vi "STC_main_raw_1.vi"() -> ()   [LabVIEW 2017]
uses:
  controls/FPGA State.ctl
  controls/UI Data2.ctl
  controls/Chatter data.ctl
  Globals/Global - All UI Loop Stop.vi
  Globals/Global - UI Stream and Variable Connections.vi
  Globals/Global - Configuration Options.vi
  UI Error Handlers/support/User Event - Stop/User Event - Stop.lvlib
  UI Error Handlers/support/Message Queue/Message Queue.lvlib
panel:
  out "resulting string":string
  out "Raw Waveform":waveform(dbl)[](graph)
  in  "Settings Tab":T1(tab)=enum."Data Monitoring"
  in  "OK Button":bool
  in  "Tool Data File":path=path "K:/Core Research/Project Folders/AI Projects/AI3190 Digital Shop Floor Rollout/5 Software Files/Catapult/tool_path.txt"
  in  "Run Control":bool
  in  "Stop Control":bool
  in  "Max Acceleration Threshold (g)":sgl=0.03
  in  "In-cut Power Threshold":dbl=1.0
  in  "Controller Address":string="172.22.11.2"
  in  "Connect to Controller":bool
  out "Connected?":bool
  out "System Status":string
  in  "Save?":bool
  in  "Switch to Safe State":bool
  out "Current FPGA State":T2
  out "Tool Data":string="\n"
  in  "ODBC data source name":string="amrc_monitoring"
  in  "MT Connect Agent":string="http://amrcmtconnect.shef.ac.uk:5000/"
  in  "milliseconds to wait":u32=100
  in  "Machine":string="STC1250"
  out "Loop execution":u32
  out "output cluster":cluster{"G1 ":bool}
  out "tag acc":string
  out "tag spike":string
  out "Chatter?":bool
  out "Feed":dbl
  out "ACC  (grms)":T3(graph)
  out "Block of code being executed":string
  out "Program Name":string
  out "RPM":dbl
  out "STC Starrag":bool
  out "Force (grms)":T4(graph)
  out "Tool id":string
  out "Spindle Load":dbl[](graph)
  out "CPU Usage (%)":dbl[][](graph)
  out "Free Physical Memory or Largest Contiguous Memory (bytes)":dbl(graph)
  out "DMA FIFO Overflow?":bool
  in  "Exit":bool
  # "Acceleration Waveform for 0.5s"
  # "Connection Settings"
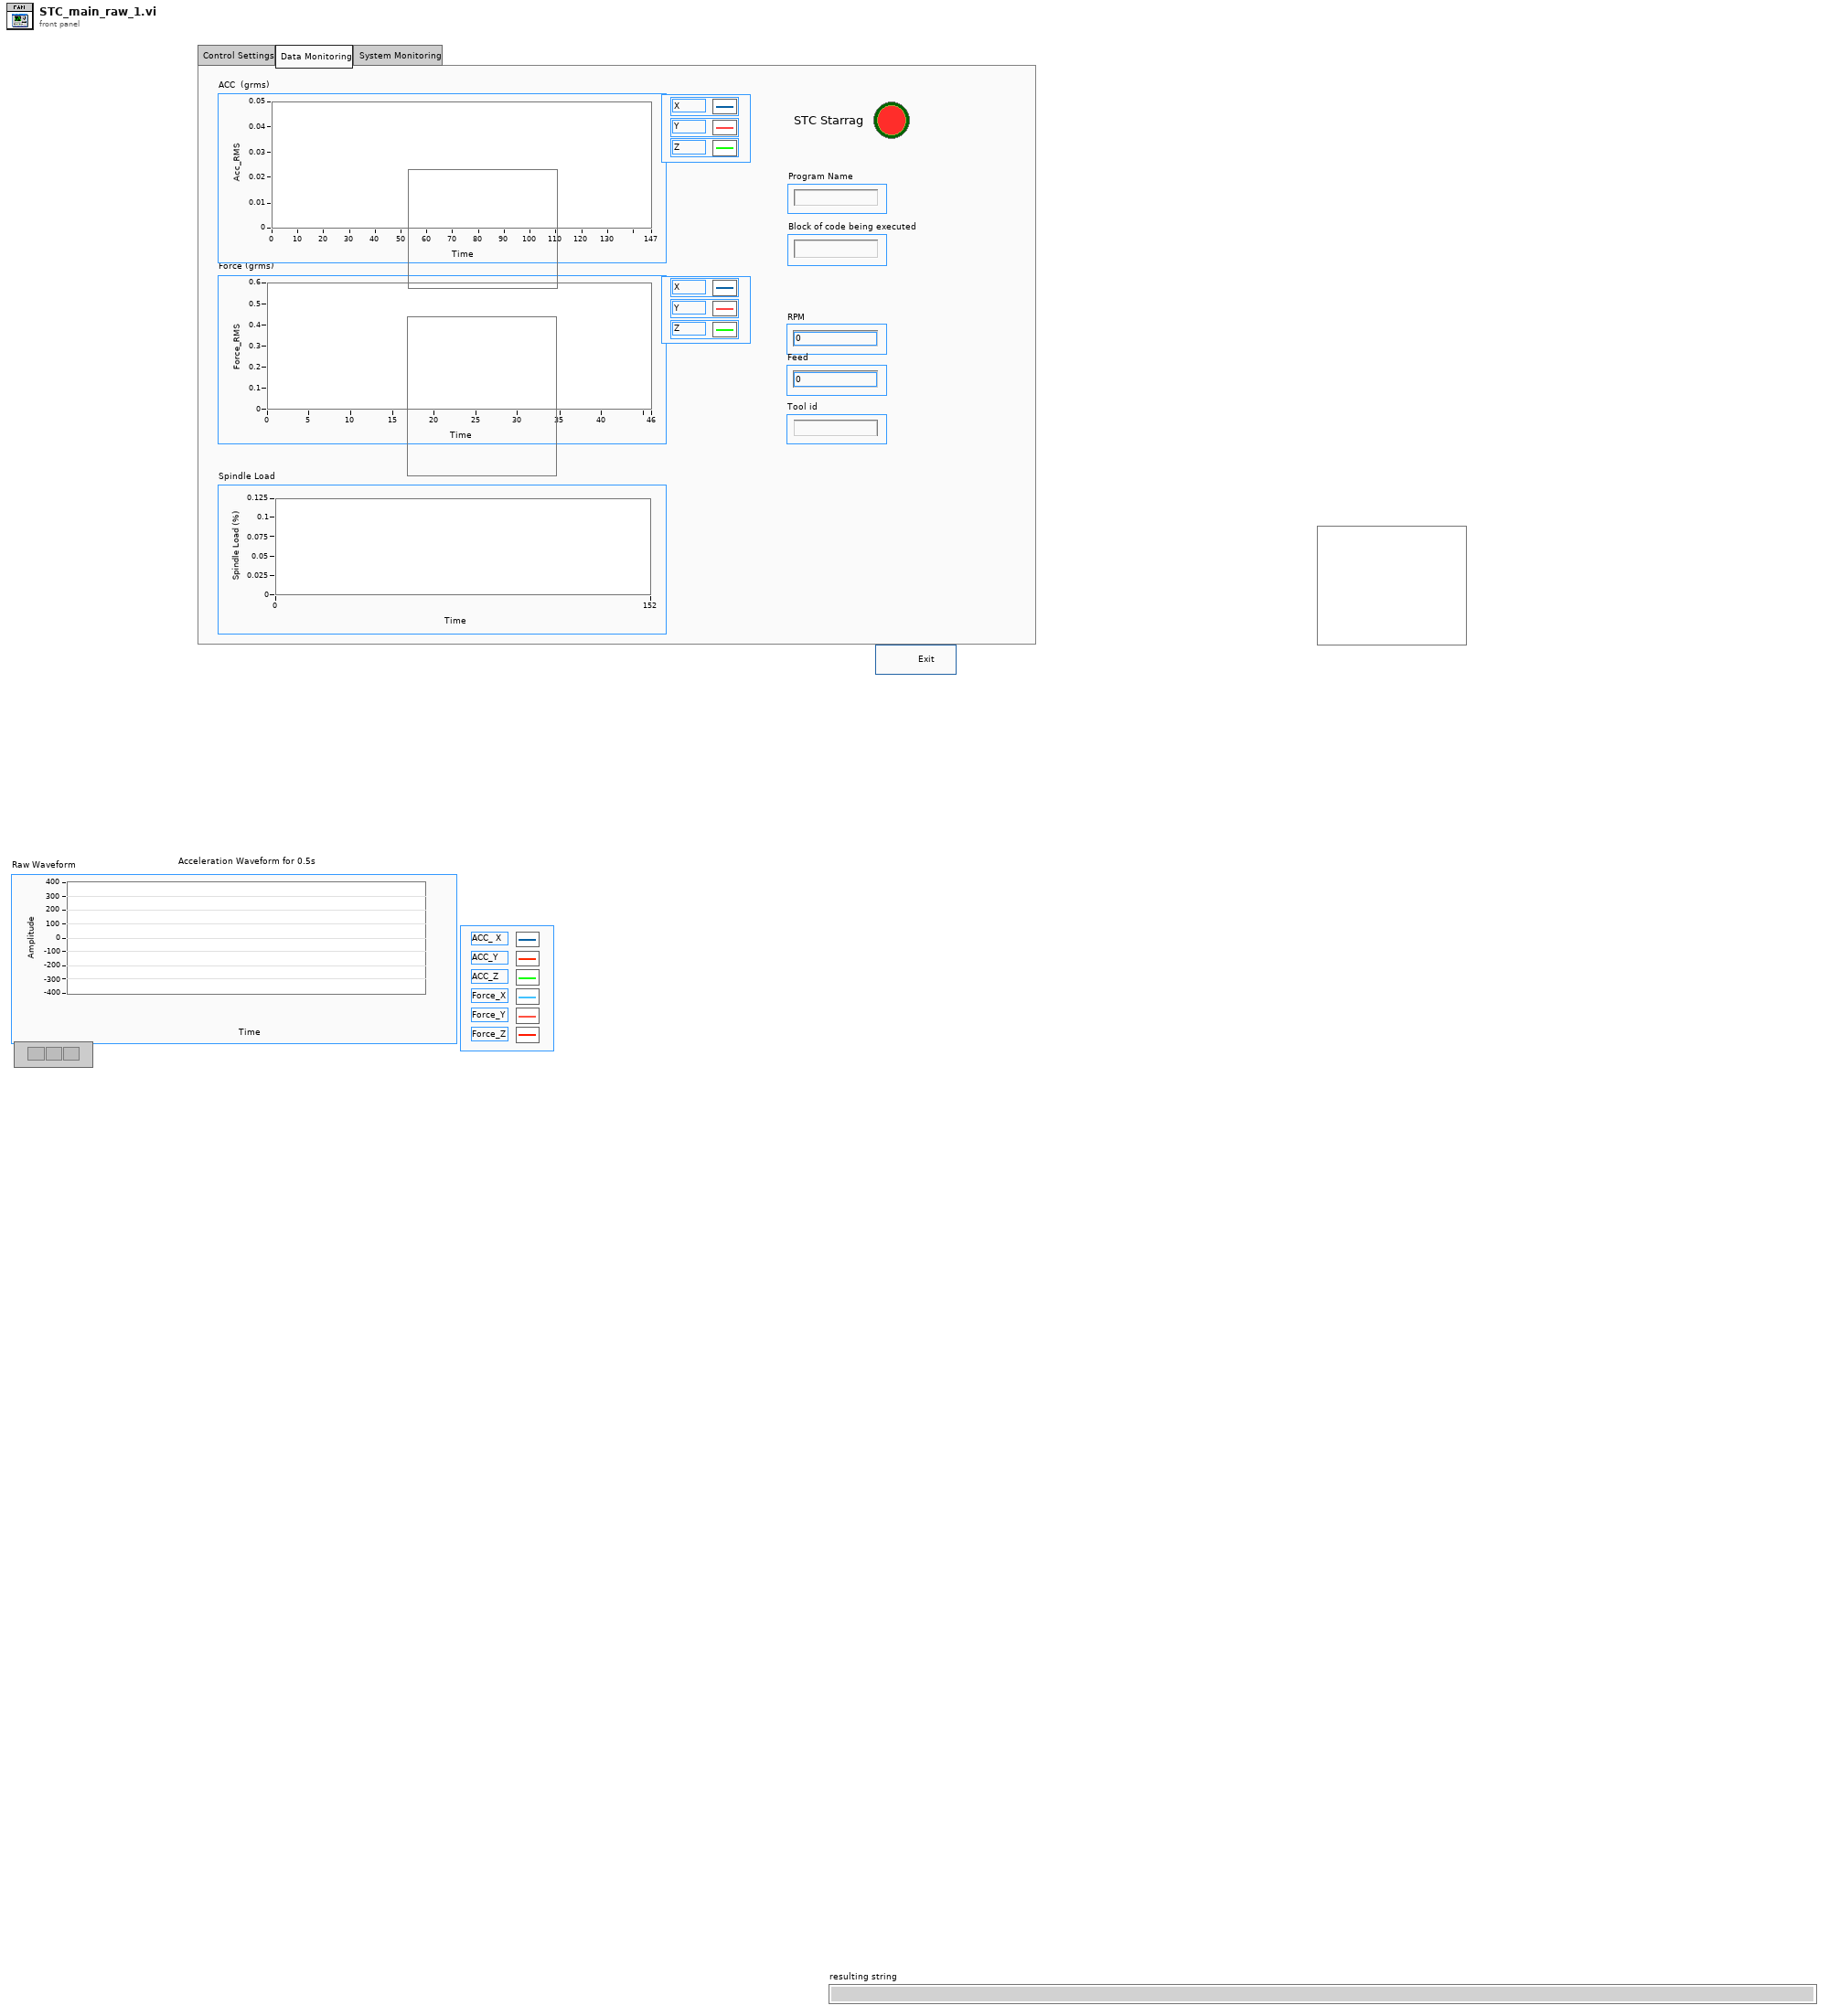
[diagram p1: front panel]
types:
  T1 = enum32{"Control Settings", "Data Monitoring", "System Monitoring"}
  T2 = typedef "FPGA State.ctl" = enum16{"Safe State", "Control (PID)"}
  T3 = cluster{"Array of Double[0]":dbl, "Array of Double[1]":dbl, "Array of Double[2]":dbl}
  T4 = cluster{"[0]":dbl, "[1]":dbl, "[2]":dbl, "[3]":dbl, "[4]":dbl, "[5]":dbl, "[6]":dbl, "[7]":dbl}
  T5 = typedef "UI Data2.ctl" = cluster{"Switch to Safe State Ref":refnum<vi>, "Run Control Ref":refnum<vi>, "Stop Control Ref":refnum<vi>, "Update Control Configurations Ref":refnum<vi>, "Chatter Data Ref":refnum<vi>, "Max Acceleration Threshold Ref":refnum<vi>}
  T6 = typedef "Message Queue.lvlib/All Message Queues.ctl" = cluster{"UI":refnum<queue>}
  T7 = enum8{"Enabled", "Disabled", "Disabled and Grayed Out"}
  T8 = cluster{"Message":string, "Message Data":variant}
  T9 = typedef "Chatter data.ctl" = cluster{"Tool data":cluster{"Number of teeth":sgl}, "Cutting data":cluster{"rpm":sgl}, "Limits":cluster{"Magnitude threshold":sgl, "Tolerance":sgl}, "G1 status":cluster{"G1 ":bool}}
  T10 = cluster{"FPGA State":T2, "Max Acceleration Threshold":sgl, "Chatter Data":T9}
  T11 = cluster{"seconds since 1Jan1904":timestamp, "number":dbl[][], "Machine Data":cluster{"Zload":string, "Yload":string, "Xload":string, "path_position":string, "Fovr":string, "SspeedOvr":string, "Program Name":string, "Program status":string, "Block of code being executed":string, "Line of code":string, "Machine availability":string, "Emergency status":string, "Controller mode":string, "Tool_id":string}}
  T12 = cluster{"seconds since 1Jan1904":timestamp, "number":dbl[][], "Machine Data":cluster{"Zload":string, "Yload":string, "Xload":string, "path_position":string, "Fovr":string, "SspeedOvr":string, "Program Name":string, "Program status":string, "Block of code being executed":string, "Line of code":string, "Machine availability":string, "Emergency status":string, "Controller mode":string, "Tool id":string}}
  T13 = cluster{"Actual PID Loop Period":refnum<k21>, "DMA FIFO Overflow?":refnum<k21>, "CPU Usage":refnum<k21>, "Free or Contiguous Memory":refnum<k21>, "Current FPGA State":refnum<k21>, "Acceleration (grms)":refnum<k21>, "Acceleration Waveform":refnum<k21>, "Chatter":refnum<k21>, "tag acc":refnum<k21>, "tag video":refnum<k21>}
  T14 = cluster{"Zload":string, "Yload":string, "Xload":string, "path_position":string, "Fovr":string, "SspeedOvr":string, "Program Name":string, "Program status":string, "Block of code being executed":string, "Line of code":string, "Machine availability":string, "Emergency status":string, "Controller mode":string, "Tool_id":string}
  T15 = cluster{"Zload":string, "Yload":string, "Xload":string, "path_position":string, "Fovr":string, "SspeedOvr":string, "Program Name":string, "Program status":string, "Block of code being executed":string, "Line of code":string, "Machine availability":string, "Emergency status":string, "Controller mode":string, "Tool id":string}
  T16 = cluster{"Magnitude threshold":sgl, "Tolerance":sgl}
  T17 = typedef "FPGA state.ctl" = enum16{"Safe State", "Control (PID)"}
  T18 = typedef "CPU Loads.ctl" = cluster{"Total (%)":dbl, "Time Critical (%)":dbl, "Timed Structures (%)":dbl, "High (%)":dbl, "Above Normal (%)":dbl, "Normal (%)":dbl, "Background (%)":dbl, "Idle (%)":dbl, "ISR (%)":dbl}[]
  T19 = cluster{"seconds since 1Jan1904":timestamp, "appended array":dbl[][], "Machine Data":cluster{"Zload":string, "Yload":string, "Xload":string, "path_position":string, "Fovr":string, "SspeedOvr":string, "Program Name":string, "Program status":string, "Block of code being executed":string, "Line of code":string, "Machine availability":string, "Emergency status":string, "Controller mode":string, "Tool_id":string}}
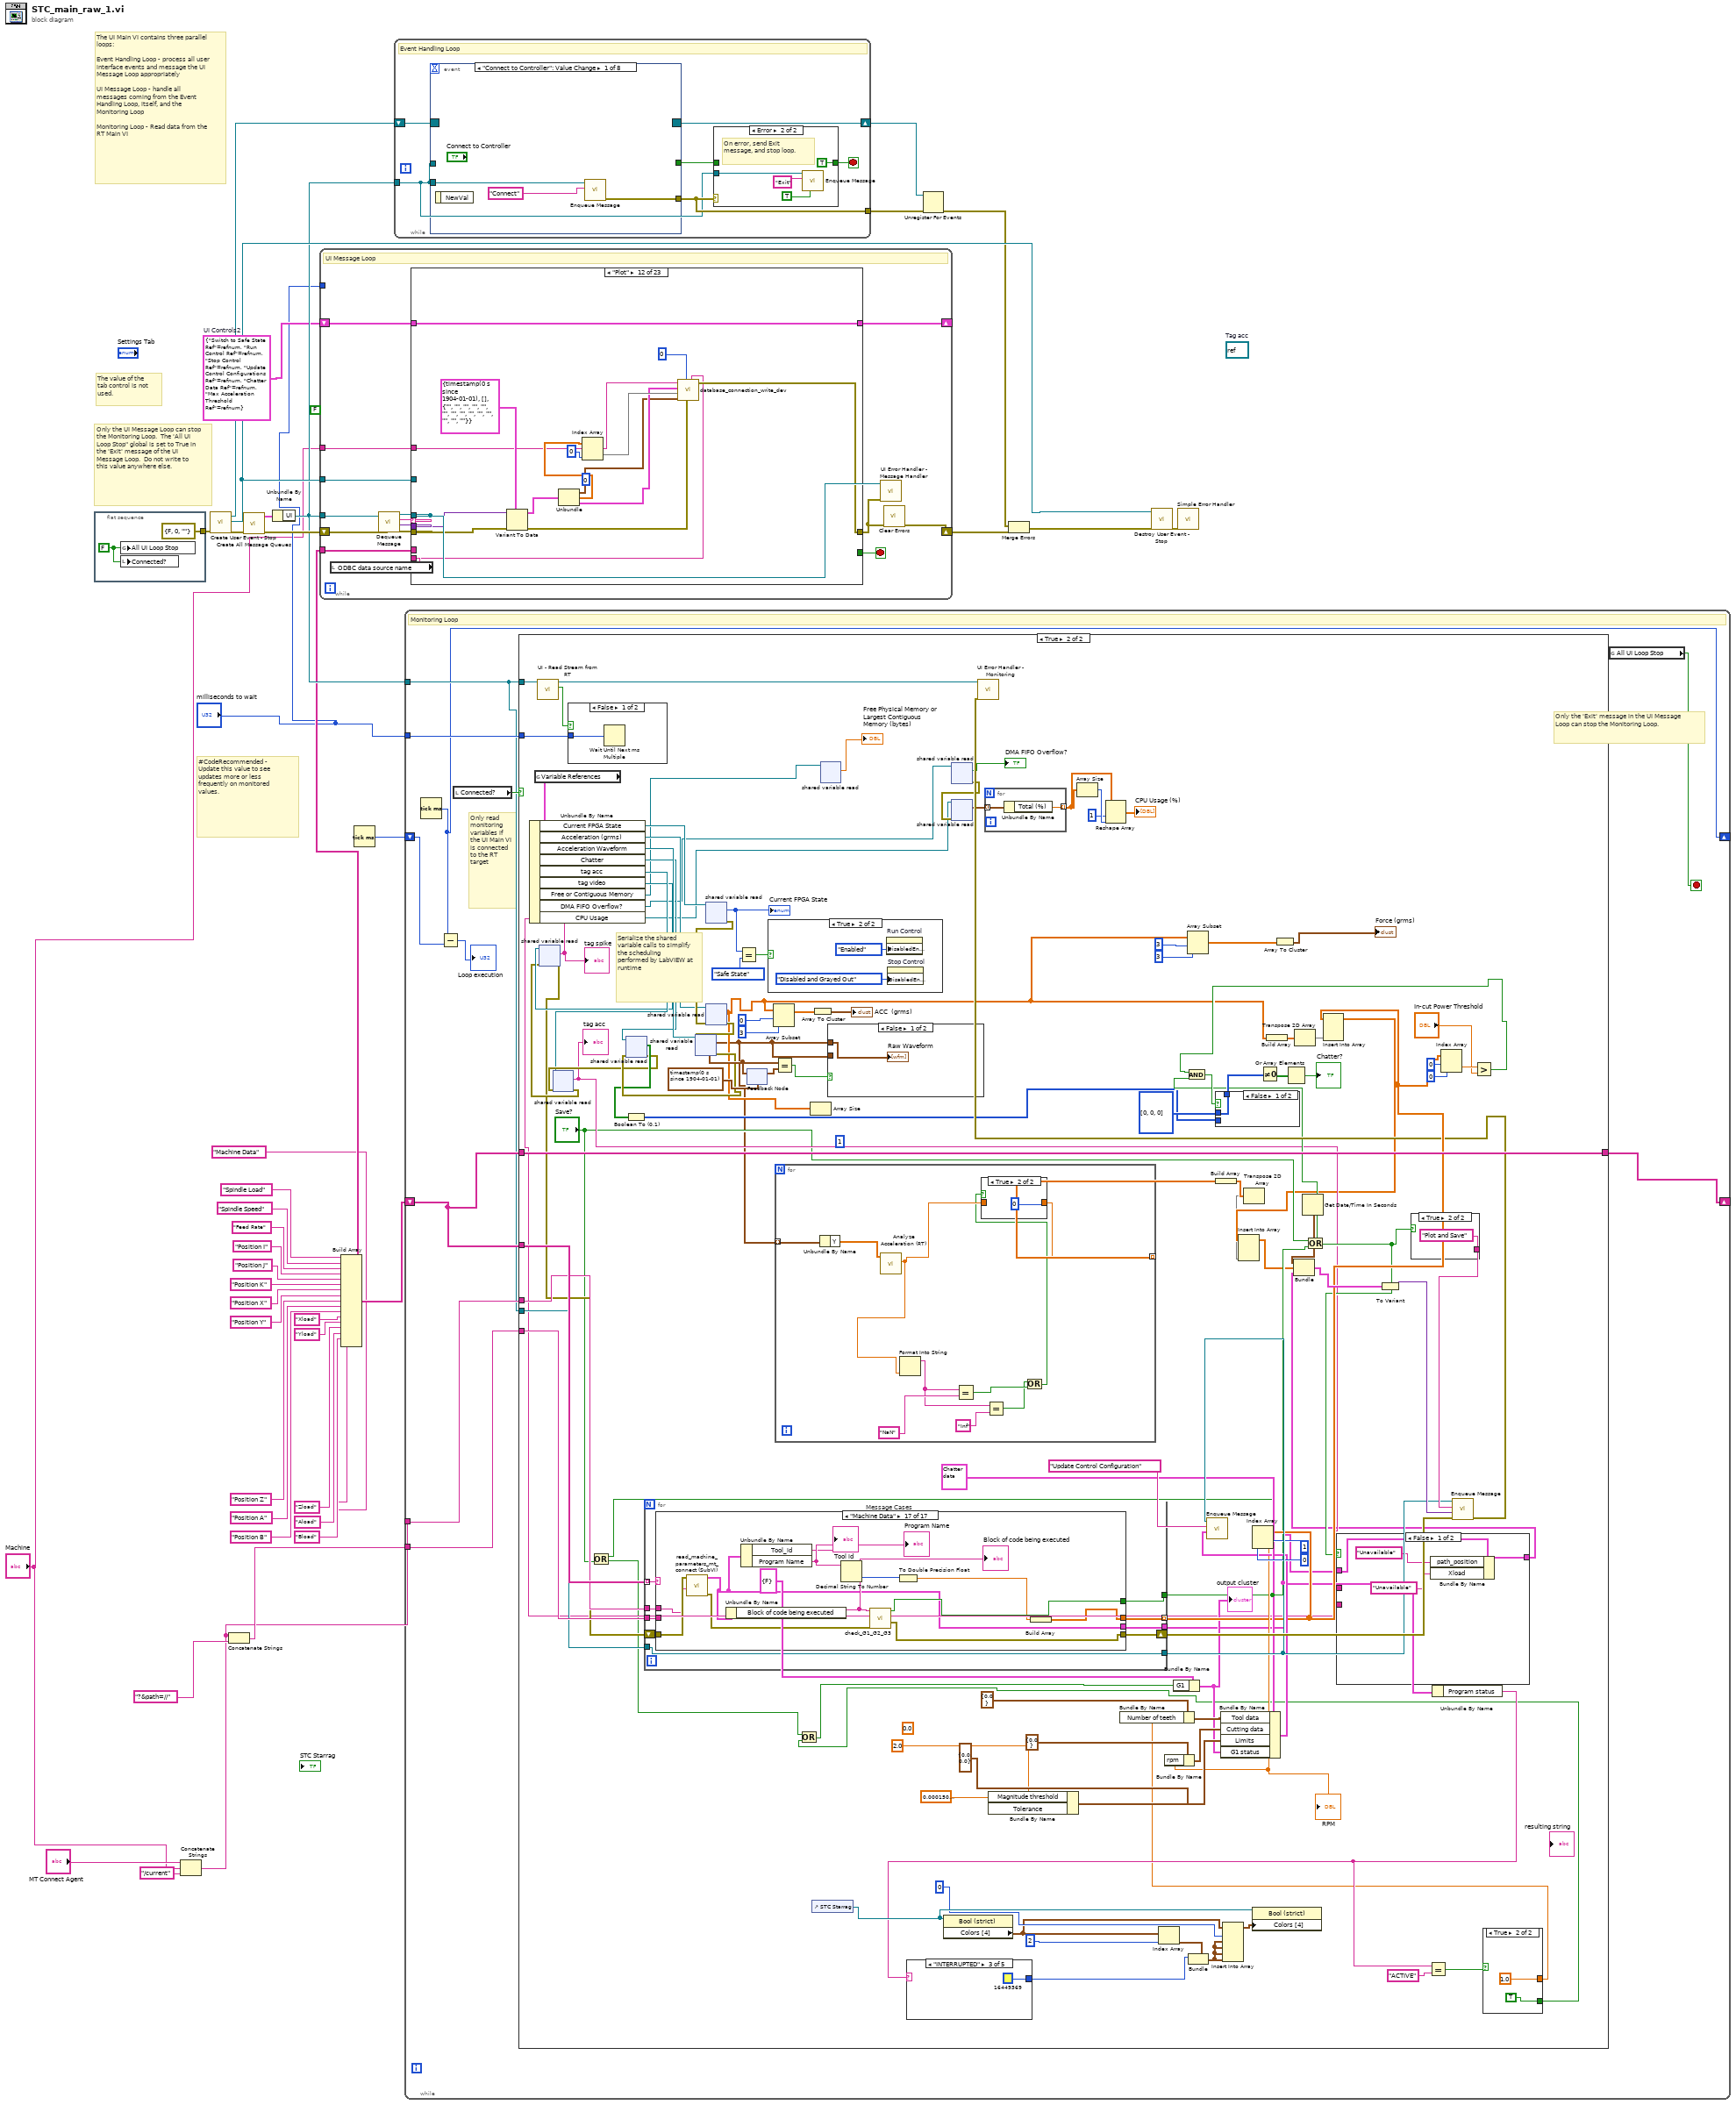
[diagram p0: block diagram]
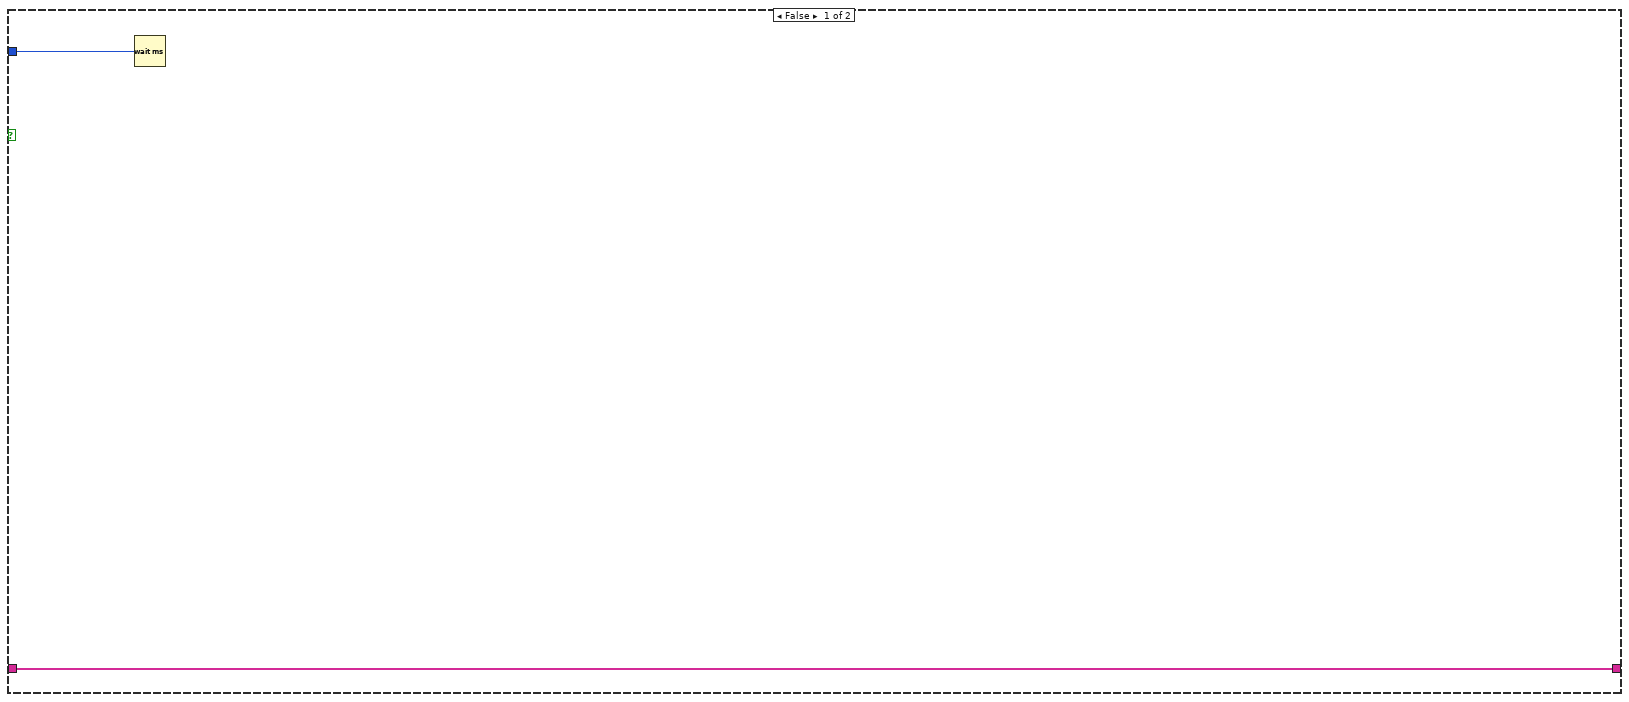
[diagram p2: hidden frame]
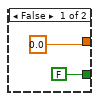
[diagram p3: hidden frame]
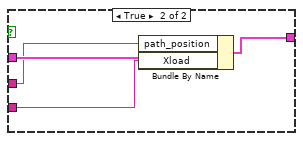
[diagram p5: hidden frame]
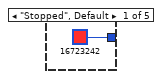
[diagram p6: hidden frame]
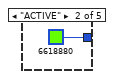
[diagram p7: hidden frame]
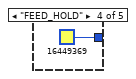
[diagram p8: hidden frame]
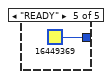
[diagram p9: hidden frame]
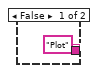
[diagram p11: hidden frame]
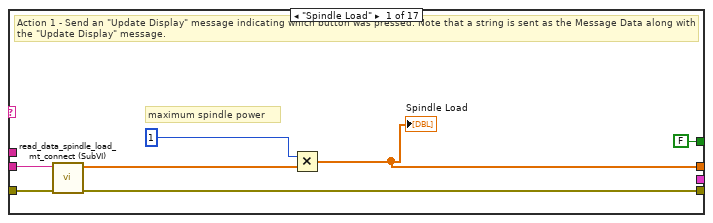
[diagram p12: hidden frame]
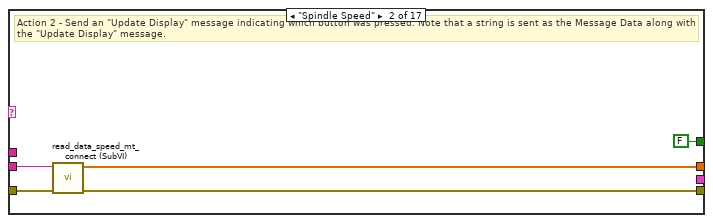
[diagram p13: hidden frame]
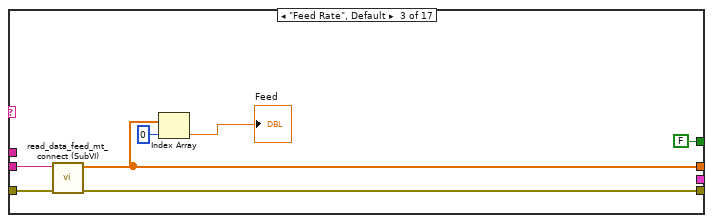
[diagram p14: hidden frame]
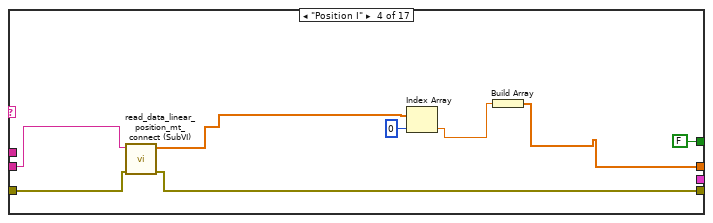
[diagram p15: hidden frame]
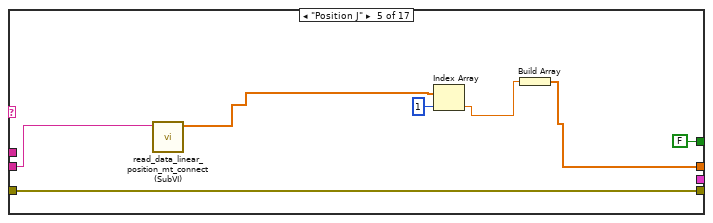
[diagram p16: hidden frame]
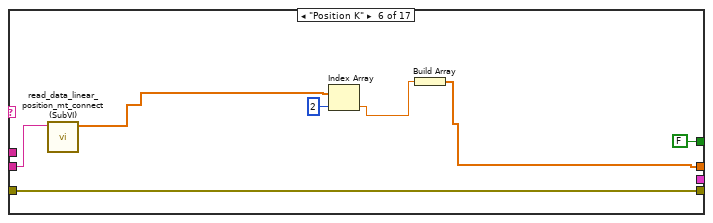
[diagram p17: hidden frame]
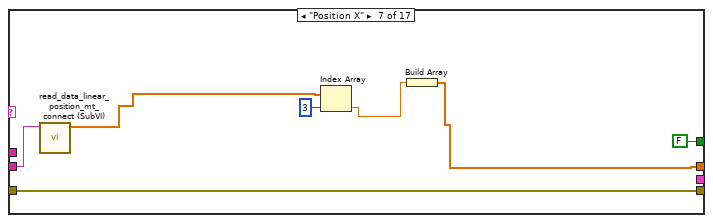
[diagram p18: hidden frame]
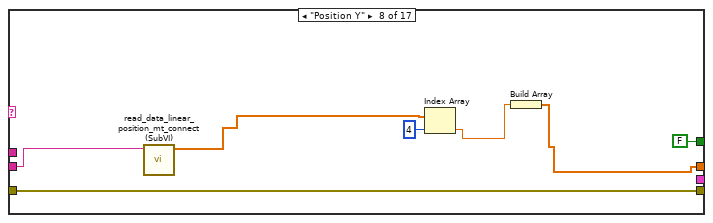
[diagram p19: hidden frame]
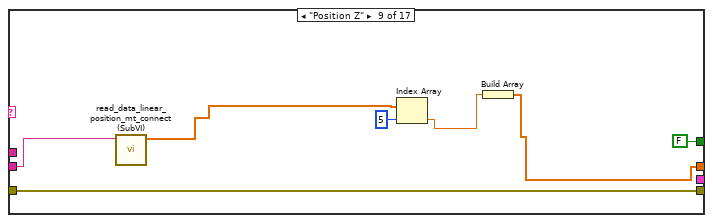
[diagram p20: hidden frame]
diagram:
  (unwired) refnum<k21> refnum  # Tag acc
  (unwired) FALSE ("Record  SS 661")
  w27 = T5 {"Switch to Safe State Ref"=refnum, "Run Control Ref"=refnum, "Stop Control Ref"=refnum, "Update Control Configurations Ref"=refnum, "Chatter Data Ref"=refnum, "Max Acceleration Threshold Ref"=refnum}  # UI Controls2
  # "#CodeRecommended - Update this value to see updates more or less frequently on monitored values."
  # "The UI Main VI contains three parallel loops:\n\nEvent Handling Loop - process all user interface events and message the UI Message Loop appropriately\n\nUI Message Loop - handle all messages coming from the Event Handling Loop, itself, and the Monitoring Loop\n\nMonitoring Loop - Read data from the RT Main VI"
  # "The value of the tab control is not used."
  # "Only the UI Message Loop can stop the Monitoring Loop.  The 'All UI Loop Stop\" global is set to True in the 'Exit' message of the UI Message Loop.  Do not write to this value anywhere else."
  n1 = flat-sequence {
    tunnel: [errorcluster {"status"=FALSE, "code"=0, "source"=""} ("error in (no error)")] -> w28
    frame #0 {
      w41 = FALSE
      n2 = global write "Global - All UI Loop Stop.vi" "All UI Loop Stop"(w41) -> ()
      n3 = local write "Connected?"(w41) -> ()
    }
  }
  n4 = Concatenate Strings("MT Connect Agent", "Machine", "/current" ("string")) -> (w18:string)
  n5 = call "Create User Event - Stop.vi"("error in (no error)"=w28) -> ("error out"=w35:errorcluster, "User Event - Stop"=w36:refnum<user-event>, "Stop Event Registration Refnum"=w37:refnum<event-registration>)  [unwired: 8 in]
  n6 = Concatenate Strings(w18, "?&path=//" ("string")) -> (w22:string)
  n7 = call "Create All Message Queues.vi"("error in (no error)"=w35) -> ("error out"=w33:errorcluster, "Message Queues out"=w34:T6)  [unwired: 9 in]
  n8 = Unbundle By Name(w34) -> ("UI"=w29:refnum<queue>)
  n9 = Build Array("Spindle Load" ("Message"), "Spindle Speed" ("Message"), "Feed Rate" ("element"), "Position I" ("element"), "Position J" ("element"), "Position K" ("element"), "Position X" ("element"), "Position Y" ("element"), "Position Z" ("element"), "Position A" ("element"), "Position B" ("element"), "Xload" ("element"), "Yload" ("element"), "Zload" ("element"), "Aload" ("element"), "Bload" ("element"), "Machine Data" ("element")) -> (w21:string[])
  n10 = while {
    tunnel: w29 -> [w51]
    tunnel: w36 -> [w56]
    shift-right: [w46] -> w40
    shift-left: w33 -> [w55]
    shift-right: [w49] -> _
    shift-left: w27 -> [w50]
    tunnel: w21 -> [w45]
    tunnel: "Machine" -> [w44]
    tunnel: "milliseconds to wait" -> [_]
    stop <- w57 stop-if-true
    # "UI Message Loop"
    n11 = local read "ODBC data source name"() -> (w43:string)
    n12 = call "Dequeue Message.vi"("error in (no error)"=w55, "Message Queue"=w51) -> ("error out"=w54:errorcluster, "Message Data"=w52:variant, "Message"=w53:string, "dup Message Queue"=w48:refnum<queue>)  [unwired: 6 in]
    n13 = case "Message Cases" shown="\"Plot\"" w53 {
      selector: w53 -> [_ _ _ _ _ _ _ _ _ _ _ _ w192 _ w226 _ w261 _ _ _ _ _ w360]
      tunnel: w48 -> [w59 w65 _ _ w98 _ w116 w124 _ w149 _ _ w193 _ _ _ w265 _ w308 _ _ w334 _]
      tunnel: w54 -> [w61 w72 w85 w91 w103 w114 w118 w122 w138 w158 w174 w189 w195 w213 w227 w245 w275 w296 w313 w318 w330 w335 _]
      tunnel: [w60 w66 w85 w91 w97 w114 w117 w127 w137 w151 w163 w177 w194 w215 w228 w244 w276 w294 w314 w317 w329 w338 w358] -> w47
      tunnel: [_ _ _ _ _ _ _ _ _ _ _ _ _ _ _ _ _ _ TRUE _ _ _ _] -> w57
      tunnel: w52 -> [_ _ _ _ _ _ _ _ _ w156 w173 w188 _ w212 w225 w243 w273 w293 _ _ w327 _ _]
      tunnel: w56 -> [_ _ _ _ _ _ _ _ _ _ _ _ _ _ _ _ _ _ w312 _ _ _ _]
      tunnel: w50 -> [w62 w71 w84 w93 w102 w113 w120 w128 w139 w154 w175 w190 w196 w216 w229 w242 w277 w295 w310 w316 w328 w337 w356]
      tunnel: [w62 w70 w84 w93 w102 w113 w120 w128 w139 w154 w175 w190 w196 w216 w229 w242 w277 w295 w310 w316 w328 w337 w356] -> w49
      tunnel: w45 -> [_ _ _ _ _ _ _ _ _ _ _ _ _ _ _ _ _ _ _ _ _ _ _]
      tunnel: w43 -> [_ _ _ _ _ _ _ _ _ _ w162 w176 _ _ _ _ _ _ _ _ _ _ _]
      tunnel: w44 -> [_ _ _ _ _ _ _ _ _ _ w167 w182 _ _ _ _ _ _ _ _ _ _ _]
      frame "Initialize" {
        # "Initialize - Send 'Initialize UI Refs' message to get the UI references bundled and initialized appropriately."
        n14 = call "Enqueue Message.vi"("error in (no error)"=w61, "Message"="Initialize UI Refs", "Message Queue"=w59) -> ("error out"=w60:errorcluster)  [unwired: 7 in, 1 out]
      }
      frame "Initialize UI Refs" {
        # "Send a message to disable them all, since there is no connection at the start."
        # "Initialize UI Refs - Bundle up a cluster of references of all UI elements that are programmatically manipulated."
        n15 = control-ref of="Max Acceleration Threshold (g)"() -> (w63:refnum<vi>)
        n16 = control-ref of="Switch to Safe State"() -> (w69:refnum<vi>)
        n17 = control-ref of="Run Control"() -> (w68:refnum<vi>)
        n18 = control-ref of="Stop Control"() -> (w67:refnum<vi>)
        n19 = call "Enqueue Message.vi"("error in (no error)"=w72, "Message"="Disable Controls", "Message Queue"=w65) -> ("error out"=w66:errorcluster)  [unwired: 7 in, 1 out]
        n20 = Bundle By Name(cluster=w71, "Switch to Safe State Ref"=w69, "Run Control Ref"=w68, "Stop Control Ref"=w67, "Max Acceleration Threshold Ref"=w63) -> (w70:T5)
      }
      frame "Disable Controls" {
        w75 = 0
        # "With the control options disabled, the only thing the user can do is Connect. Make sure the IP address string and connect button are enabled."
        # "Disable All Controls - Set all controls in the UI Refs cluster to \"Disabled and Grayed Out\"."
        n21 = Unbundle(w84) -> ("Switch to Safe State Ref"=w83:refnum<vi>, "Run Control Ref"=w82:refnum<vi>, "Stop Control Ref"=w81:refnum<vi>, "Update Control Configurations Ref"=w80:refnum<vi>, "Chatter Data Ref"=w79:refnum<vi>, "Max Acceleration Threshold Ref"=w78:refnum<vi>)
        n22 = Build Array(w83, w82, w81, w80, w79, w78) -> (w77:refnum<vi>[])
        n23 = property on="ODBC data source name" class="Str"("DisabledEnum"=T7."Enabled" ("Disabled")) -> ()  [unwired: 2 in, 2 out]
        n24 = property on="In-cut Power Threshold" class="DigNum (strict)"("DisabledEnum"=T7."Disabled and Grayed Out" ("Disabled")) -> ()  [unwired: 2 in, 2 out]
        n25 = call "Set Enable State on Multiple Controls.vi"("Enable?"=FALSE, "Controls"=w77) -> ()  [unwired: 10 in]
        n26 = property on="Controller Address" class="Str"("DisabledEnum"=w75) -> ()  [unwired: 2 in, 2 out]
        n27 = property on="Connect to Controller" class="Bool"("DisabledEnum"=w75) -> ()  [unwired: 2 in, 2 out]
      }
      frame "Enable Configuration Controls" {
        w94 = 2
        # "Once connected, the user shouldn't be able to change the connection settings unless he gets disconnected."
        # "Enable Configuration Controls - After successful connection, ensure appropriate controls are enabled."
        n28 = Unbundle By Name(w93) -> ("Update Control Configurations Ref"=w92:refnum<vi>, "Max Acceleration Threshold Ref"=w90:refnum<vi>, "Chatter Data Ref"=w89:refnum<vi>, "Switch to Safe State Ref"=w88:refnum<vi>)
        n29 = property on="In-cut Power Threshold" class="DigNum (strict)"("DisabledEnum"=T7."Enabled" ("Disabled")) -> ()  [unwired: 2 in, 2 out]
        n30 = property on="ODBC data source name" class="Str"("DisabledEnum"=T7."Disabled and Grayed Out" ("Disabled")) -> ()  [unwired: 2 in, 2 out]
        n31 = Build Array(w92, w90, w89, w88) -> (w96:refnum<vi>[])
        n32 = call "Set Enable State on Multiple Controls.vi"("Enable?"=TRUE, "Controls"=w96) -> ()  [unwired: 10 in]
        n33 = property on="Controller Address" class="Str"("DisabledEnum"=w94) -> ()  [unwired: 2 in, 2 out]
        n34 = property on="Connect to Controller" class="Bool"("DisabledEnum"=w94) -> ()  [unwired: 2 in, 2 out]
      }
      frame "Connect" {
        # "Connect - Attempt to connect to both streams, and the variables, on the RT target."
        n35 = call "UI - Initiate Connection.vi"("error in (no error)"=w103, "Controller Address"="Controller Address", "Message Queue"=w98) -> ("error out"=w100:errorcluster, "Connected?"=w99:bool)  [unwired: 7 in]
        "Connected?" <- w99
        n36 = case shown="True" w99 {
          tunnel: w100 -> [w104 w108]
          tunnel: w98 -> [_ w107]
          tunnel: [w104 w106] -> w97
          frame False {
          }
          frame True {
            n37 = call "Enqueue Message.vi"("error in (no error)"=w108, "Message"="Enable Configuration Controls", "Message Queue"=w107) -> ("error out"=w106:errorcluster)  [unwired: 7 in, 1 out]
          }
        }
      }
      frame "Close Connections" {
        # "Close Connections - Close the connections shared with the Monitoring Loop."
        n38 = global read "Global - UI Stream and Variable Connections.vi" "UI Command Stream"() -> (w112:refnum<k21>)
        n39 = global read "Global - UI Stream and Variable Connections.vi" "RT Message Stream"() -> (w111:refnum<k21>)
        n40 = global read "Global - UI Stream and Variable Connections.vi" "Variable References"() -> (w109:T13)
        n41 = local write "Connected?"(FALSE ("Connected?")) -> ()
        n42 = Destroy Stream Endpoint(11:w112) -> ()  [unwired: 1 in, 1 out]
        n43 = Destroy Stream Endpoint(11:w111) -> ()  [unwired: 1 in, 1 out]
        n44 = call "Close Variable Connections.vi"("Variable References 2"=w109) -> ()  [unwired: 11 in]
      }
      frame "Disconnect UI" {
        # "Disable Controls"
        # "Disconnect UI - Something has gone wrong with the connection. Reinitialize the UI to its disconnected state."
        n45 = local write "Connected?"(FALSE ("Connected?")) -> ()
        n46 = call "Enqueue Message.vi"("error in (no error)"=w118, "Message"="Reconnect", "Message Queue"=w116) -> ("error out"=w117:errorcluster)  [unwired: 7 in, 1 out]
      }
      frame "Reconnect" {
        # "Disconnect UI - Something has gone wrong with the connection. Reinitialize the UI to its disconnected state."
        n47 = Flush Queue(queue=w124, error in (no error)=w122) -> (queue out=w123:refnum<queue>, error out=w121:errorcluster)  [unwired: 1 out]
        n48 = flat-sequence {
          tunnel: w123 -> [w130]
          tunnel: w121 -> [w131]
          tunnel: [w131] -> w126
          tunnel: [w130] -> w125
          tunnel: w126 -> [w134]
          tunnel: w125 -> [w132]
          tunnel: [w133] -> w127
          frame #0 {
            n49 = Wait Until Next ms Multiple(millisecond multiple=u32 10000) -> ()  [unwired: 1 out]
          }
          frame #1 {
            n50 = call "Enqueue Message.vi"("error in (no error)"=w134, "Message"="Connect", "Message Queue"=w132) -> ("error out"=w133:errorcluster)  [unwired: 7 in, 1 out]
          }
        }
      }
      frame "Get Settings from FPGA" {
        # "Get Settings from FPGA - Send a command to the RT to retrieve all current FPGA Main VI parameter values and send them back to the UI."
        n51 = local read "Connected?"() -> (w136:bool)
        n52 = case shown="True" w136 {
          tunnel: w138 -> [w140 w144]
          tunnel: [w140 w143] -> w137
          frame False {
            # "Don't bother trying to send a message to the RT system if UI Main VI isn't even connected"
          }
          frame True {
            n53 = global read "Global - UI Stream and Variable Connections.vi" "UI Command Stream"() -> (w141:refnum<k21>)
            n54 = shared-variable-write(w141, w144, T8 {"Message"="Send FPGA Configuration to UI", "Message Data"=variant} ("data in")) -> (w143:errorcluster)  [unwired: 1 in, 2 out]
          }
        }
      }
      frame "Initial UI Values" {
        # "Set values of all manual and setpoint controls via reference."
        # "Initial UI Values - These are the current values of the FPGA Main VI's R/W controls. They are used to initialize the panel of UI Main VI upon successful connection to the RT target."
        n55 = Variant To Data(error in=w158, type=T10 {"FPGA State"=enum."Safe State", "Max Acceleration Threshold"=0.0, "Chatter Data"={"Tool data"={"Number of teeth"=2.0}, "Cutting data"={"rpm"=9898.0}, "Limits"={"Magnitude threshold"=0.0, "Tolerance"=1.0}, "G1 status"={"G1 "=FALSE}}}, Variant=w156) -> (data=w155:T10, error out=w157:errorcluster)
        n56 = Unbundle By Name(w154) -> ("Max Acceleration Threshold Ref"=w146:refnum<vi>)
        n57 = Unbundle By Name(w155) -> ("Max Acceleration Threshold"=w148:sgl, "FPGA State"=w147:T2)  [unwired: 1 out]
        n58 = Build Array(w146, w146) -> (w153:refnum<vi>[])
        n59 = Build Array(w148) -> (w152:sgl[])
        n60 = for {
          tunnel: w153 -> [w160] mode=indexing
          tunnel: w152 -> [w159] mode=indexing
          n61 = property class="DigNum (strict)"(reference=w160, "Value"=w159) -> ()  [unwired: 1 in, 2 out]
        }
        n62 = local write "Current FPGA State"(w147) -> ()
        n63 = call "Enqueue Message.vi"("error in (no error)"=w157, "Message Data"=w147, "Message"="Update Display Mode", "Message Queue"=w149) -> ("error out"=w151:errorcluster)  [unwired: 6 in, 1 out]
      }
      frame "Plot and Save" {
        n64 = Variant To Data(error in=w174, type=T11 {"seconds since 1Jan1904"=timestamp(0 s since 1904-01-01), "number"=[], "Machine Data"={"Zload"="", "Yload"="", "Xload"="", "path_position"="", "Fovr"="", "SspeedOvr"="", "Program Name"="", "Program status"="", "Block of code being executed"="", "Line of code"="", "Machine availability"="", "Emergency status"="", "Controller mode"="", "Tool_id"=""}} ("output cluster"), Variant=w173) -> (data=w172:T11, error out=w164:errorcluster)
        n65 = Unbundle(w172) -> ("seconds since 1Jan1904"=w165:timestamp, "number"=w170:dbl[][], "Machine Data"=w168:T14)
        n66 = Index Array(array=w170, index (col)=0 ("disabled index (col)")) -> (element=w161:dbl[])  [unwired: 1 in]
        n67 = call "database_connection_write_dev.vi"("ODBC data source name"=w162, "error in (no error)"=w164, "G1?"=u32 1, "current time"=w165, "data 2"=w161, "Machine Data"=w168, "Machine type"=w167) -> ("error out"=w163:errorcluster)  [unwired: 4 in]
      }
      frame "Plot" {
        (unwired) u32 0 ("G1?")
        n68 = Variant To Data(error in=w189, type=T12 {"seconds since 1Jan1904"=timestamp(0 s since 1904-01-01), "number"=[], "Machine Data"={"Zload"="", "Yload"="", "Xload"="", "path_position"="", "Fovr"="", "SspeedOvr"="", "Program Name"="", "Program status"="", "Block of code being executed"="", "Line of code"="", "Machine availability"="", "Emergency status"="", "Controller mode"="", "Tool id"=""}} ("output cluster"), Variant=w188) -> (data=w186:T12, error out=w178:errorcluster)
        n69 = Unbundle(w186) -> ("seconds since 1Jan1904"=w180:timestamp, "number"=w184:dbl[][], "Machine Data"=w181:T15)
        n70 = Index Array(array=w184, index (col)=0 ("disabled index (col)")) -> (element=w183:dbl[])  [unwired: 1 in]
        n71 = call "database_connection_write_dev.vi"("ODBC data source name"=w176, "error in (no error)"=w178, "G1?"=u32 0, "current time"=w180, "data 2"=w183, "Machine Data"=w181, "Machine type"=w182) -> ("error out"=w177:errorcluster)  [unwired: 4 in]
      }
      frame "Run Control", "Run Safe State", "Stop Control" {
        # "Run/Stop buttons - Send a command to switch the FPGA into the appropriate state. Send a message to update this UI to reflect the new state."
        n72 = local read "Connected?"() -> (w191:bool)
        n73 = case shown="False" w191 {
          tunnel: w195 -> [w197 w207]
          tunnel: [w197 w203] -> w194
          tunnel: w193 -> [_ w202]
          tunnel: w192 -> [_ w201]
          frame False {
            # "Don't bother trying to send a message to the RT system if UI Main VI isn't even connected"
          }
          frame True {
            # "Run Control switch into Run Control state. Anything else switches to Safe State."
            n74 = case shown="\"Run Control\"" w201 {
              tunnel: [FPGA_State."Safe State" ("FPGA State") FPGA_State."Control (PID)" ("FPGA State")] -> w198
              frame "Safe State", "Stop Control", Default {
              }
              frame "Run Control" {
              }
            }
            n75 = global read "Global - UI Stream and Variable Connections.vi" "UI Command Stream"() -> (w199:refnum<k21>)
            n76 = Bundle("Update FPGA State", "FPGA State"=w198) -> (w204:cluster{string, "FPGA State":T2})  [unwired: 1 in]
            n77 = shared-variable-write(w199, w207, w204) -> (w206:errorcluster)  [unwired: 1 in, 2 out]
            n78 = call "Enqueue Message.vi"("error in (no error)"=w206, "Message Data"=w198, "Message"="Update Display Mode", "Message Queue"=w202) -> ("error out"=w203:errorcluster)  [unwired: 6 in, 1 out]
          }
        }
      }
      frame "Update Control Configuration" {
        # "Update Control Configuration - Send all control configurations to RT to be sent down to the FPGA."
        n79 = Variant To Data(type=T9 {"Tool data"={"Number of teeth"=2.0}, "Cutting data"={"rpm"=9898.0}, "Limits"={"Magnitude threshold"=0.0, "Tolerance"=1.0}, "G1 status"={"G1 "=FALSE}} ("Chatter Data"), Variant=w212) -> (data=w211:T9)  [unwired: 1 in, 1 out]
        n80 = local read "Connected?"() -> (w214:bool)
        n81 = case shown="True" w214 {
          tunnel: w213 -> [w217 w223]
          tunnel: [w217 w222] -> w215
          tunnel: w211 -> [_ w218]
          frame False {
            # "Don't bother trying to send a message to the RT system if UI Main VI isn't even connected"
          }
          frame True {
            n82 = global read "Global - UI Stream and Variable Connections.vi" "UI Command Stream"() -> (w219:refnum<k21>)
            n83 = Bundle("Update Control Configurations", "Chatter Data"=w218) -> (w220:cluster{string, "Chatter Data":T9})  [unwired: 1 in]
            n84 = shared-variable-write(w219, w223, w220) -> (w222:errorcluster)  [unwired: 1 in, 2 out]
          }
        }
      }
      frame "Update Max Acceleration Threshold", "Update Max Fan Speed Threshold", "Update Setpoints" {
        # "Update Manual Values/Setpoints - Send all manual values/setpoints to RT to be sent down to the FPGA."
        n85 = local read "Connected?"() -> (w224:bool)
        n86 = case shown="True" w224 {
          tunnel: [w230 w236] -> w228
          tunnel: w227 -> [w230 w234]
          tunnel: w226 -> [_ w233]
          tunnel: w225 -> [_ w232]
          frame False {
            # "Don't bother trying to send a message to the RT system if UI Main VI isn't even connected"
          }
          frame True {
            n87 = global read "Global - UI Stream and Variable Connections.vi" "UI Command Stream"() -> (w231:refnum<k21>)
            n88 = Bundle(w233, "Message Data"=w232) -> (w235:cluster{string, "Message Data":variant})  [unwired: 1 in]
            n89 = shared-variable-write(w231, w234, w235) -> (w236:errorcluster)  [unwired: 1 in, 2 out]
          }
        }
      }
      frame "Update Display Mode" {
        # "Update Display Mode - Enable/Disable Controls appropriately for the new display mode."
        n90 = Variant To Data(error in=w245, type=FPGA_State."Safe State" ("FPGA State"), Variant=w243) -> (data=w241:T2, error out=w244:errorcluster)
        n91 = Unbundle By Name(w242) -> ("Switch to Safe State Ref"=w240:refnum<vi>, "Stop Control Ref"=w238:refnum<vi>, "Run Control Ref"=w237:refnum<vi>)
        n92 = case shown="\"Control (PID)\"" w241 {
          tunnel: w240 -> [w248 w254]
          tunnel: w237 -> [w246 w255]
          tunnel: w238 -> [w247 w253]
          frame "Control (PID)" {
            n93 = Build Array "Controls to Enable"(w248, w247) -> (w252:refnum<vi>[])
            n94 = Build Array "Controls to Disable"(w246) -> (w250:refnum<vi>[])
            n95 = call "Set Enable State on Multiple Controls.vi"("Enable?"=FALSE, "Controls"=w250) -> ()  [unwired: 10 in]
            n96 = call "Set Enable State on Multiple Controls.vi"("Enable?"=TRUE, "Controls"=w252) -> ()  [unwired: 10 in]
          }
          frame "Safe State", Default {
            # "This frame runs when FPGA is in Safe State. Only enable the run button."
            n97 = Build Array "Controls to Enable"(w255) -> (w259:refnum<vi>[])
            n98 = Build Array "Controls to Disable"(w254, w253) -> (w257:refnum<vi>[])
            n99 = call "Set Enable State on Multiple Controls.vi"("Enable?"=FALSE, "Controls"=w257) -> ()  [unwired: 10 in]
            n100 = call "Set Enable State on Multiple Controls.vi"("Enable?"=TRUE, "Controls"=w259) -> ()  [unwired: 10 in]
          }
        }
      }
      frame "Critical Error", "Log-Only Error", "Non-Critical Error", "RT Error" {
        # "Error - Display message in status indicator on panel.  If it's a critical error, shut down this VI with an 'Exit' message."
        n101 = case shown="Default" w261 {
          selector: w261 -> [_ w279]
          tunnel: ["UI Error" w279] -> w260
          frame Default {
          }
          frame "RT Error" {
          }
        }
        n102 = Variant To Data(error in=w275, type=errorcluster {"status"=FALSE, "code"=0, "source"=""} ("error constant"), Variant=w273) -> (data=w268:errorcluster, error out=w274:errorcluster)
        n103 = Unbundle By Name(w268) -> ("code"=w267:i32, "source"=w271:string)
        n104 = Format Date/Time String() -> (date/time string=w270:string)  [unwired: 3 in]
        n105 = Format Into String(format string="\n%s: %s %d - %s", w270, w260, w267, w271) -> (resulting string=w262:string)  [unwired: 2 in, 1 out]
        n106 = call "Enqueue Message.vi"("error in (no error)"=w274, "Message Data"=w262, "Message"="Update System Status", "Message Queue"=w265) -> ("error out"=w266:errorcluster, "dup Message Queue"=w264:refnum<queue>)  [unwired: 6 in]
        n107 = case shown="Default" w261 {
          tunnel: w266 -> [w280 w284]
          tunnel: w264 -> [_ w282]
          tunnel: [w280 w283] -> w276
          frame Default {
          }
          frame "Critical Error" {
            n108 = call "Enqueue Message.vi"("error in (no error)"=w284, "Message"="Exit", "Message Queue"=w282) -> ("error out"=w283:errorcluster)  [unwired: 7 in, 1 out]
          }
        }
      }
      frame "Update System Status" {
        # "#CodeRecommended - The code below ensures that the System Status string value does not become too large.  It uses the same maximum size as the RT error log to determine whether or not to remove the last half of the log string. Change this logic if you wish to maintain more/less of the information in the System Status string."
        # "Update System Status - Add a new string to the beginning of the System Status string on the UI."
        n109 = Variant To Data(error in=w296, type="", Variant=w293) -> (data=w290:string, error out=w294:errorcluster)
        n110 = local read "System Status"() -> (w288:string)
        n111 = global read "Global - Configuration Options.vi" "Error Log Max Size (bytes)"() -> (w286:i64)
        n112 = String Length(string=w288) -> (length=w289:i32)
        n113 = Greater?(x=w289, y=w286) -> (0:w287:bool)
        n114 = case shown="False" w287 {
          tunnel: w288 -> [w297 w301]
          tunnel: w286 -> [_ w300]
          tunnel: [w297 w302] -> w285
          frame False {
          }
          frame True {
            n115 = Divide(x=w300, y=i64 2) -> (x/y=w299:dbl)
            n116 = String Subset(string=w301, length (rest)=w299) -> (substring=w302:string)  [unwired: 1 in]
          }
        }
        n117 = Concatenate Strings(w290, w285) -> (→"System Status":string)
      }
      frame "Exit" {
        # "Close all connections"
        # "Stop Monitoring Loop"
        # "Stop Event Handling Loop"
        # "Release the UI Message queue reference"
        # "Stop UI Message Loop"
        # "Exit - Fire the User Event to stop the Event Handling Loop, and toggle the local variable to stop the Monitoring Loop.  This message alone causes all three loops to stop."
        n118 = local write "Connected?"(FALSE ("Connected?")) -> ()
        n119 = global write "Global - All UI Loop Stop.vi" "All UI Loop Stop"(TRUE ("Stop Monitoring Loop")) -> ()
        n120 = call "Fire User Event - Stop.vi"("User Event - Stop"=w312) -> ("error out"=w311:errorcluster)  [unwired: 10 in]
        n121 = Release Queue(queue=w308, error in (no error)=w313) -> (error out=w309:errorcluster)  [unwired: 1 in, 2 out]
        n122 = global read "Global - UI Stream and Variable Connections.vi" "UI Command Stream"() -> (w307:refnum<k21>)
        n123 = global read "Global - UI Stream and Variable Connections.vi" "RT Message Stream"() -> (w306:refnum<k21>)
        n124 = global read "Global - UI Stream and Variable Connections.vi" "Variable References"() -> (w303:T13)
        n125 = Destroy Stream Endpoint(11:w307) -> ()  [unwired: 1 in, 1 out]
        n126 = Destroy Stream Endpoint(11:w306) -> ()  [unwired: 1 in, 1 out]
        n127 = call "Close Variable Connections.vi"("Variable References 2"=w303) -> ()  [unwired: 11 in]
        n128 = Merge Errors(w311, w309) -> (w314:errorcluster)
      }
      frame "---Copy This Frame---" {
        # "Duplicate this frame when creating new messages.  Change this comment in the duplicated frame to describe this message."
        n129 = Merge Errors(w318) -> (w317:errorcluster)
      }
      frame "Update Tool Data" {
        # "Duplicate this frame when creating new messages.  Change this comment in the duplicated frame to describe this message."
        n130 = Variant To Data(type=path "" ("Tool Data File"), Variant=w327) -> (data=w319:path, error out=w321:errorcluster)  [unwired: 1 in]
        n131 = Build Path(name or relative path=w319) -> (appended path=w325:path)  [unwired: 1 in]
        n132 = Read from Text File(file (use dialog)=w325, error in=w321) -> (text=w322:string, error out=w324:errorcluster)  [unwired: 2 in, 2 out]
        n133 = Unbundle By Name(w324) -> ("status"=w323:bool)  [unwired: 1 out]
        n134 = case shown="False" w323 {
          tunnel: w322 -> [w331 _]
          tunnel: [w331 "Error"] -> w320
          frame False {
          }
          frame True {
          }
        }
        "Tool Data" <- w320
        n135 = Merge Errors(w330) -> (w329:errorcluster)
      }
      frame "Unsuccessful Connection" {
        # "Duplicate this frame when creating new messages.  Change this comment in the duplicated frame to describe this message."
        n136 = flat-sequence {
          tunnel: w337 -> [w340]
          tunnel: [w340] -> w336
          tunnel: w336 -> [w341]
          tunnel: w335 -> [w354]
          tunnel: [w353] -> w333
          tunnel: w334 -> [w352]
          frame #0 {
            n137 = local write "Connected?"(FALSE ("Connected?")) -> ()
          }
          frame #1 {
            w342 = 0
            n138 = Unbundle(w341) -> ("Switch to Safe State Ref"=w350:refnum<vi>, "Run Control Ref"=w349:refnum<vi>, "Stop Control Ref"=w348:refnum<vi>, "Update Control Configurations Ref"=w347:refnum<vi>, "Chatter Data Ref"=w346:refnum<vi>, "Max Acceleration Threshold Ref"=w345:refnum<vi>)
            n139 = property on="Controller Address" class="Str"("DisabledEnum"=w342) -> ()  [unwired: 2 in, 2 out]
            n140 = property on="Connect to Controller" class="Bool"("DisabledEnum"=w342) -> ()  [unwired: 2 in, 2 out]
            n141 = Build Array(w350, w349, w348, w347, w346, w345) -> (w344:refnum<vi>[])
            n142 = call "Set Enable State on Multiple Controls.vi"("Enable?"=FALSE, "Controls"=w344) -> ()  [unwired: 10 in]
          }
          frame #2 {
            n143 = Wait (ms)(milliseconds to wait=u32 1000) -> ()  [unwired: 1 out]
          }
          frame #3 {
            n144 = call "Enqueue Message.vi"("error in (no error)"=w354, "Message"="Connect", "Message Queue"=w352) -> ("error out"=w353:errorcluster)  [unwired: 7 in, 1 out]
          }
        }
        n145 = Merge Errors(w333) -> (w338:errorcluster)
      }
      frame Default {
        # "'Default' case only runs if there is a message that isn't defined in any of the other cases.  Output a programming error."
        n146 = Format Into String(format string="The invalid message string \"%s\" was received in the Message Handling Loop." ("Invalid Message Loop Message"), w360) -> (resulting string=w357:string)  [unwired: 2 in, 1 out]
        n147 = call <vilib>:"Error Cluster From Error Code.vi"("error message (\"\")"=w357, "error code (0)"=1) -> ("error out"=w358:errorcluster)  [unwired: 7 in]
      }
    }
    n148 = call "UI Error Handler - Message Handler.vi"("error in (no error)"=w47, "Message Queue"=w48) -> ()  [unwired: 9 in, 1 out]
    n149 = call <vilib>:"Clear Errors.vi"("error in (no error)"=w47) -> ("error out"=w46:errorcluster)  [unwired: 5 in, 1 out]
  }
  n150 = Tick Count (ms)() -> (millisecond timer value=w17:u32)
  n151 = while {
    tunnel: w29 -> [w362]
    tunnel: [w365] -> w39
    shift-right: [w363] -> w31
    shift-left: w37 -> [w364]
    stop <- w366 stop-if-true
    # "Event Handling Loop"
    n152 = event shown="[0] \"Connect to Controller\": Value Change" {
      selector: w364 -> [_ _ _ _ _ _ _ _]
      dyn-events: [_ _ _ _ _ _ _ _] -> w363
      timeout: _ -> [_ _ _ _ _ _ _ _]
      tunnel: [_ _ _ _ _ _ _ TRUE ("Discard?")] -> w367
      tunnel: w362 -> [w373 w376 w379 w382 w387 _ w392 _]
      tunnel: [w375 w378 w381 w384 w386 _ w395 _] -> w365
      tunnel: w362 -> [_ _ _ _ _ w391 _ _]
      event "Connect to Controller": Value Change {
        n153 = event-data() -> ()  [unwired: 1 in, 1 out]
        n154 = call "Enqueue Message.vi"("Message"="Connect", "Message Queue"=w373) -> ("error out"=w375:errorcluster)  [unwired: 8 in, 1 out]
      }
      event "Run Control": Value Change {
        n155 = event-data() -> ()  [unwired: 1 in, 1 out]
        n156 = call "Enqueue Message.vi"("Message"="Run Control", "Message Queue"=w376) -> ("error out"=w378:errorcluster)  [unwired: 8 in, 1 out]
      }
      event "Stop Control": Value Change {
        n157 = event-data() -> ()  [unwired: 1 in, 1 out]
        n158 = call "Enqueue Message.vi"("Message"="Stop Control", "Message Queue"=w379) -> ("error out"=w381:errorcluster)  [unwired: 8 in, 1 out]
      }
      event "Switch to Safe State": Value Change {
        n159 = event-data() -> ()  [unwired: 1 in, 1 out]
        n160 = call "Enqueue Message.vi"("Message"="Run Safe State", "Message Queue"=w382) -> ("error out"=w384:errorcluster)  [unwired: 8 in, 1 out]
      }
      event "Max Acceleration Threshold (g)": Value Change {
        n161 = event-data() -> ()  [unwired: 1 in, 1 out]
        n162 = call "Enqueue Message.vi"("Message Data"="Max Acceleration Threshold (g)", "Message"="Update Max Acceleration Threshold", "Message Queue"=w387) -> ("error out"=w386:errorcluster)  [unwired: 7 in, 1 out]
      }
      event "Tool Data File", "OK Button": Value Change {
        n163 = event-data() -> ()  [unwired: 1 in, 3 out]
        n164 = call "Enqueue Message.vi"("Message Data"="Tool Data File", "Message"="Update Tool Data", "Message Queue"=w391) -> ()  [unwired: 7 in, 2 out]
      }
      event "Exit": Value Change {
        w393 = TRUE  # Priority Message
        # "The UI Message Loop handles sending the Exit message to other loops."
        n165 = event-data() -> ()  [unwired: 1 in, 1 out]
        n166 = call "Enqueue Message.vi"("Priority Message? (F)"=w393, "Message"="Exit", "Message Queue"=w392) -> ("error out"=w395:errorcluster)  [unwired: 7 in, 1 out]
      }
      event User Event {
        # "The Message Handling Loop processed an \"Exit\" message, which fired this event to stop the Event Handling Loop."
        n167 = event-data() -> ()  [unwired: 1 in, 1 out]
      }
    }
    n168 = case shown="Error" w365 {
      tunnel: [w368 TRUE ("Discard?")] -> w366
      tunnel: w367 -> [w368 _]
      tunnel: w362 -> [_ w369]
      frame No Error {
      }
      frame Error {
        # "On error, send Exit message, and stop loop."
        n169 = call "Enqueue Message.vi"("Priority Message? (F)"=TRUE ("Discard?"), "Message"="Exit", "Message Queue"=w369) -> ()  [unwired: 7 in, 2 out]
      }
    }
  }
  n170 = while {
    tunnel: w29 -> [w400]
    tunnel: "milliseconds to wait" -> [w405]
    shift-right: [w401] -> _
    shift-left: w21 -> [w402]
    tunnel: w18 -> [w404]
    tunnel: w22 -> [w403]
    shift-right: [w397] -> _
    shift-left: w17 -> [w399]
    stop <- w407 stop-if-true
    # "Only read monitoring variables if the UI Main VI is connected to the RT target"
    # "Only the 'Exit' message in the UI Message Loop can stop the Monitoring Loop."
    # "Monitoring Loop"
    n171 = Tick Count (ms)() -> (millisecond timer value=w397:u32)
    n172 = Subtract(x=w397, y=w399) -> (x-y=→"Loop execution":u32)
    n173 = local read "Connected?"() -> (w406:bool)
    n174 = case shown="True" w406 {
      tunnel: w400 -> [_ w524]
      tunnel: w405 -> [w409 w520]
      tunnel: w402 -> [_ w505]
      tunnel: w404 -> [_ w504]
      tunnel: w403 -> [_ w503]
      tunnel: [w408 w502] -> w401
      tunnel: w402 -> [w408 w502]
      tunnel: w400 -> [_ w501]
      frame False {
        n175 = Wait (ms)(milliseconds to wait=w409) -> ()  [unwired: 1 out]
      }
      frame True {
        (unwired) 1 ("length")
        (unwired) sgl 0.0 ("Tolerance")
        # "Serialize the shared variable calls to simplify the scheduling performed by LabVIEW at runtime"
        n176 = global read "Global - UI Stream and Variable Connections.vi" "Variable References"() -> (w522:T13)
        n177 = Unbundle By Name(w522) -> ("Current FPGA State"=w519:refnum<k21>, "Acceleration (grms)"=w516:refnum<k21>, "Acceleration Waveform"=w515:refnum<k21>, "Chatter"=w442:refnum<k21>, "tag acc"=w450:refnum<k21>, "tag video"=w449:refnum<k21>, "Free or Contiguous Memory"=w420:refnum<k21>, "DMA FIFO Overflow?"=w419:refnum<k21>, "CPU Usage"=w418:refnum<k21>)
        n178 = call "UI - Read Stream from RT.vi"("Message Queue"=w524) -> ("Message Received?"=w521:bool, "dup Message Queue"=w523:refnum<queue>)  [unwired: 8 in, 1 out]
        n179 = case shown="False" w521 {
          tunnel: w520 -> [w697 _]
          frame False {
            n180 = Wait Until Next ms Multiple(millisecond multiple=w697) -> ()  [unwired: 1 out]
          }
          frame True {
            # "If a message was received, immediately read again"
          }
        }
        n181 = shared-variable-read(w519) -> (w518:errorcluster, w508:T17)  [unwired: 1 in, 2 out]
        "Current FPGA State" <- w508
        n182 = shared-variable-read(w516, w518) -> (w517:errorcluster, w443:dbl[])  [unwired: 2 out]
        n183 = shared-variable-read(w515, w517) -> (w495:errorcluster, w433:waveform(dbl)[], w512:timestamp)  [unwired: 1 out]
        n184 = shared-variable-read(w442, w495) -> (w451:errorcluster, w494:bool[])  [unwired: 2 out]
        n185 = shared-variable-read(w450, w451) -> (w448:errorcluster, w440:string)  [unwired: 2 out]
        "tag acc" <- w440
        n186 = shared-variable-read(w449, w448) -> (w447:errorcluster, w436:string)  [unwired: 2 out]
        "tag spike" <- w436
        n187 = Boolean To (0,1)(Boolean=w494) -> (0, 1=w434:i16[])
        n188 = for {
          tunnel: w505 -> [w566] mode=indexing
          shift-right: [w568] -> w500
          shift-left: w447 -> [w567]
          tunnel: [w560] -> w478 mode=indexing
          tunnel: [w565] -> w492
          tunnel: w501 -> [w565]
          tunnel: w503 -> [w564]
          tunnel: w504 -> [w563]
          tunnel: [w561] -> w446
          tunnel: [w562] -> w438
          n189 = case "Message Cases" shown="\"Machine Data\"" w566 {
            tunnel: w567 -> [w575 w580 w587 w594 w602 w609 w616 w623 w630 w637 w644 w651 w658 w665 w672 w679 w684]
            tunnel: [w574 w579 w586 w592 w602 w609 w616 w623 w630 w637 w644 w651 w658 w665 w672 w679 w690] -> w568
            tunnel: [w569 w578 w583 w588 w597 w604 w611 w618 w625 w632 w640 w646 w654 w660 w667 w676 w680] -> w560
            tunnel: w564 -> [w571 w577 w585 w593 w598 w605 w612 w619 w626 w633 w638 w650 w652 w664 w668 w674 _]
            tunnel: w563 -> [_ _ _ _ _ _ _ _ _ _ _ _ _ _ _ _ w683]
            tunnel: [FALSE ("Triggger G1,G2, or G3") FALSE ("Triggger G1,G2, or G3") FALSE ("Triggger G1,G2, or G3") FALSE ("Triggger G1,G2, or G3") FALSE ("Triggger G1,G2, or G3") FALSE ("Triggger G1,G2, or G3") FALSE ("Triggger G1,G2, or G3") FALSE ("Triggger G1,G2, or G3") FALSE ("Triggger G1,G2, or G3") FALSE ("Triggger G1,G2, or G3") FALSE ("Triggger G1,G2, or G3") FALSE ("Triggger G1,G2, or G3") FALSE ("Triggger G1,G2, or G3") FALSE ("Triggger G1,G2, or G3") FALSE ("Triggger G1,G2, or G3") FALSE ("Triggger G1,G2, or G3") w689] -> w561
            tunnel: [_ _ _ _ _ _ _ _ _ _ _ _ _ _ _ _ w681] -> w562
            frame "Spindle Load" {
              # "maximum spindle power"
              # "Action 1 - Send an \"Update Display\" message indicating which button was pressed. Note that a string is sent as the Message Data along with the \"Update Display\" message."
              n190 = call "read_data_spindle_load_mt_connect (SubVI).vi"("error in (no error)"=w575, "URL"=w571) -> ("error out"=w574:errorcluster, "number"=w572:dbl[])  [unwired: 8 in]
              n191 = Multiply(x=1, y=w572) -> (x*y=w569:dbl[])
              "Spindle Load" <- w569
            }
            frame "Spindle Speed" {
              # "Action 2 - Send an \"Update Display\" message indicating which button was pressed. Note that a string is sent as the Message Data along with the \"Update Display\" message."
              n192 = call "read_data_speed_mt_connect (SubVI).vi"("error in (no error)"=w580, "URL"=w577) -> ("error out"=w579:errorcluster, "number"=w578:dbl[])  [unwired: 8 in]
            }
            frame "Feed Rate", Default {
              n193 = call "read_data_feed_mt_connect (SubVI).vi"("error in (no error)"=w587, "URL"=w585) -> ("error out"=w586:errorcluster, "appended array"=w583:dbl[])  [unwired: 8 in]
              n194 = Index Array(array=w583, index=0) -> (element=→"Feed":dbl)
            }
            frame "Position I" {
              n195 = call "read_data_linear_position_mt_connect (SubVI).vi"("error in (no error)"=w594, "URL"=w593) -> ("error out"=w592:errorcluster, "I, J,K,X, Y,Z"=w590:dbl[])  [unwired: 8 in]
              n196 = Index Array(array=w590, index=0) -> (element=w589:dbl)
              n197 = Build Array(w589) -> (w588:dbl[])
            }
            frame "Position J" {
              n198 = call "read_data_linear_position_mt_connect (SubVI).vi"("URL"=w598) -> ("I, J,K,X, Y,Z"=w600:dbl[])  [unwired: 9 in, 1 out]
              n199 = Index Array(array=w600, index=1) -> (element=w599:dbl)
              n200 = Build Array(w599) -> (w597:dbl[])
            }
            frame "Position K" {
              n201 = call "read_data_linear_position_mt_connect (SubVI).vi"("URL"=w605) -> ("I, J,K,X, Y,Z"=w607:dbl[])  [unwired: 9 in, 1 out]
              n202 = Index Array(array=w607, index=2) -> (element=w606:dbl)
              n203 = Build Array(w606) -> (w604:dbl[])
            }
            frame "Position X" {
              n204 = call "read_data_linear_position_mt_connect (SubVI).vi"("URL"=w612) -> ("I, J,K,X, Y,Z"=w614:dbl[])  [unwired: 9 in, 1 out]
              n205 = Index Array(array=w614, index=3) -> (element=w613:dbl)
              n206 = Build Array(w613) -> (w611:dbl[])
            }
            frame "Position Y" {
              n207 = call "read_data_linear_position_mt_connect (SubVI).vi"("URL"=w619) -> ("I, J,K,X, Y,Z"=w621:dbl[])  [unwired: 9 in, 1 out]
              n208 = Index Array(array=w621, index=4) -> (element=w620:dbl)
              n209 = Build Array(w620) -> (w618:dbl[])
            }
            frame "Position Z" {
              n210 = call "read_data_linear_position_mt_connect (SubVI).vi"("URL"=w626) -> ("I, J,K,X, Y,Z"=w628:dbl[])  [unwired: 9 in, 1 out]
              n211 = Index Array(array=w628, index=5) -> (element=w627:dbl)
              n212 = Build Array(w627) -> (w625:dbl[])
            }
            frame "Position A" {
              n213 = call "read_data_linear_angle_mt_connect (SubVI).vi"("URL"=w633) -> ("I, J,K,X, Y,Z"=w635:dbl[])  [unwired: 9 in, 1 out]
              n214 = Index Array(array=w635, index=0) -> (element=w634:dbl)
              n215 = Build Array(w634) -> (w632:dbl[])
            }
            frame "Position B" {
              n216 = call "read_data_linear_angle_mt_connect (SubVI).vi"("URL"=w638) -> ("I, J,K,X, Y,Z"=w642:dbl[])  [unwired: 9 in, 1 out]
              n217 = Index Array(array=w642, index=1) -> (element=w641:dbl)
              n218 = Build Array(w641) -> (w640:dbl[])
            }
            frame "Xload" {
              n219 = call "read_data_linear_loadX_mt_connect (SubVI).vi"("URL"=w650) -> ("I, J,K,X, Y,Z"=w648:dbl[])  [unwired: 9 in, 1 out]
              n220 = Index Array(array=w648, index=0) -> (element=w647:dbl)
              n221 = Build Array(w647) -> (w646:dbl[])
            }
            frame "Yload" {
              n222 = call "read_data_linear_loadX_mt_connect (SubVI).vi"("URL"=w652) -> ("I, J,K,X, Y,Z"=w656:dbl[])  [unwired: 9 in, 1 out]
              n223 = Index Array(array=w656, index=1) -> (element=w655:dbl)
              n224 = Build Array(w655) -> (w654:dbl[])
            }
            frame "Zload" {
              n225 = call "read_data_linear_loadX_mt_connect (SubVI).vi"("URL"=w664) -> ("I, J,K,X, Y,Z"=w661:dbl[])  [unwired: 9 in, 1 out]
              n226 = Index Array(array=w661, index=2) -> (element=w662:dbl)
              n227 = Build Array(w662) -> (w660:dbl[])
            }
            frame "Aload" {
              n228 = call "read_data_angle_loadmt_connect (SubVI).vi"("URL"=w668) -> ("I, J,K,X, Y,Z"=w670:dbl[])  [unwired: 9 in, 1 out]
              n229 = Index Array(array=w670, index=0) -> (element=w669:dbl)
              n230 = Build Array(w669) -> (w667:dbl[])
            }
            frame "Bload" {
              n231 = call "read_data_angle_loadmt_connect (SubVI).vi"("URL"=w674) -> ("I, J,K,X, Y,Z"=w673:dbl[])  [unwired: 9 in, 1 out]
              n232 = Index Array(array=w673, index=1) -> (element=w678:dbl)
              n233 = Build Array(w678) -> (w676:dbl[])
            }
            frame "Machine Data" {
              n234 = call "read_machine_parameters_mt_connect (SubVI).vi"("URL 2"=w683, "error in (no error) 3"=w684) -> ("error out 3"=w682:errorcluster, "Machine Data"=w681:T14)  [unwired: 7 in]
              n235 = Unbundle By Name(w681) -> ("Block of code being executed"=w691:string)
              "Block of code being executed" <- w691
              n236 = Unbundle By Name(w681) -> ("Tool_id"=→"Tool id":string, "Program Name"=w688:string)
              "Program Name" <- w688
              n237 = Decimal String To Number(string=w688) -> (number=w687:i32)  [unwired: 2 in, 1 out]
              n238 = call "check_G1_G2_G3.vi"("current line"=w691, "error in (no error)"=w682) -> ("Triggger G1,G2, or G3"=w689:bool, "error out (no error)"=w690:errorcluster)  [unwired: 7 in]
              n239 = To Double Precision Float(number=w687) -> (double precision float=w686:dbl)
              n240 = Build Array(w686) -> (w680:dbl[])
            }
          }
        }
        n241 = Or(x=w446, y="Save?") -> (x .or. y?=w412:bool)
        n242 = Equal?(x=w508, y=FPGA_state."Safe State") -> (x = y?=w510:bool)
        n243 = feedback #1(timestamp(0 s since 1904-01-01)) -> (w514:timestamp)
        n244 = feedback-in #1(w512) -> ()
        n245 = case shown="True" w510 {
          frame False {
            n246 = property on="Run Control" class="Bool"("DisabledEnum"=T7."Disabled and Grayed Out" ("Disabled")) -> ()  [unwired: 2 in, 2 out]
            n247 = property on="Stop Control" class="Bool"("DisabledEnum"=T7."Enabled" ("Disabled")) -> ()  [unwired: 2 in, 2 out]
          }
          frame True {
            n248 = property on="Run Control" class="Bool"("DisabledEnum"=T7."Enabled" ("Disabled")) -> ()  [unwired: 2 in, 2 out]
            n249 = property on="Stop Control" class="Bool"("DisabledEnum"=T7."Disabled and Grayed Out" ("Disabled")) -> ()  [unwired: 2 in, 2 out]
          }
        }
        n250 = Array Subset(array=w443, index=0, length=3) -> (w444:dbl[])
        n251 = Equal?(x=w512, y=w514) -> (x = y?=w445:bool)
        n252 = for {
          tunnel: w433 -> [w540] mode=indexing
          tunnel: [w538] -> w432 mode=indexing
          n253 = Unbundle By Name(w540) -> ("Y"=w539:dbl[])
          n254 = call "Analyze Acceleration (RT).vi"("Acceleration Waveform (SGL)"=w539) -> ("Acceleration (grms)"=w536:dbl)  [unwired: 8 in, 2 out]
          n255 = Format Into String(w536) -> (resulting string=w533:string)  [unwired: 3 in, 1 out]
          n256 = Equal?(x=w533, y="NaN") -> (x = y?=w535:bool)
          n257 = Equal?(x=w533, y="Inf") -> (x = y?=w532:bool)
          n258 = Or(x=w532, y=w535) -> (x .or. y?=w531:bool)
          n259 = case shown="True" w531 {
            tunnel: [w541 0] -> w538
            tunnel: w536 -> [w541 _]
            frame False {
            }
            frame True {
            }
          }
        }
        n260 = Array Size(array=w443) -> ()  [unwired: 1 out]
        n261 = Array To Cluster(array=w444) -> (cluster=→"ACC  (grms)":cluster{"[0]":dbl, "[1]":dbl, "[2]":dbl})
        n262 = control-ref of="STC Starrag"() -> (w471:refnum<vi>)
        n263 = shared-variable-read(w420) -> (→"Free Physical Memory or Largest Contiguous Memory (bytes)":dbl)  [unwired: 1 in, 3 out]
        n264 = case shown="False" w445 {
          tunnel: w433 -> [_ _]
          tunnel: w433 -> [w696 _]
          frame False {
            "Raw Waveform" <- w696
          }
          frame True {
          }
        }
        n265 = property on="Property Node" class="Bool (strict)"(reference=w471) -> ("Colors [4]"=w465:cluster{u32, u32}[])  [unwired: 1 in, 2 out]
        n266 = shared-variable-read(w419) -> (w426:errorcluster, →"DMA FIFO Overflow?":bool)  [unwired: 1 in, 2 out]
        n267 = shared-variable-read(w418, w426) -> (w425:T18)  [unwired: 3 out]
        n268 = for {
          tunnel: w425 -> [w530] mode=indexing
          tunnel: [w529] -> w424 mode=indexing
          n269 = Unbundle By Name(w530) -> ("Total (%)"=w529:dbl)
        }
        n270 = Bundle By Name(cluster=T16 {"Magnitude threshold"=0.0, "Tolerance"=0.0} ("Limits"), "Magnitude threshold"=sgl 0.00015, "Tolerance"=sgl 2.0) -> (w484:T16)
        n271 = Array Size(array=w424) -> (size(s)=w423:i32)
        n272 = Reshape Array(w424, 1 ("dimension size"), w423) -> (→"CPU Usage (%)":dbl[][])
        n273 = Index Array(array=w465, index=2) -> (element=w467:cluster{u32, u32})
        n274 = Array Subset(array=w443, index=3, length=3) -> (w454:dbl[])
        n275 = Build Array(w432) -> (w431:dbl[][])
        n276 = Transpose 2D Array(2D array=w431) -> (transposed array=w429:dbl[][])
        n277 = Index Array(array=w478, index (row)=1, index (col)=0 ("disabled index (col)")) -> (element=w479:dbl)
        "RPM" <- w479
        n278 = Bundle By Name(cluster=cluster{"rpm":sgl} {"rpm"=0.0} ("Cutting data"), "rpm"=w479) -> (w486:cluster{"rpm":sgl})
        n279 = Build Array(w443) -> (w497:dbl[][])
        n280 = Array To Cluster(array=w454) -> (cluster=→"Force (grms)":T4)
        n281 = Transpose 2D Array(2D array=w497) -> (transposed array=w496:dbl[][])
        n282 = Get Date/Time In Seconds() -> (seconds since 1Jan1904=w506:timestamp)
        n283 = Or(x="Save?", y=w446) -> (x .or. y?=w441:bool)
        n284 = Insert Into Array(array=w478, new element=w496) -> (w430:dbl[][])  [unwired: 2 in]
        n285 = Insert Into Array(array=w430, new element=w429) -> (w428:dbl[][])  [unwired: 2 in]
        n286 = case shown="False" w441 {
          tunnel: w440 -> [_ w547]
          tunnel: [w545 w550] -> w439
          tunnel: w438 -> [w546 w549]
          tunnel: w436 -> [_ w548]
          frame False {
            n287 = Bundle By Name(cluster=w546, "path_position"="Unavailable" ("Tool_id"), "Xload"="Unavailable" ("Tool_id")) -> (w545:T14)
          }
          frame True {
            n288 = Bundle By Name(cluster=w549, "path_position"=w547, "Xload"=w548) -> (w550:T14)
          }
        }
        n289 = Bundle("seconds since 1Jan1904"=w506, "appended array"=w428, "Machine Data"=w439) -> (w507:T19)  [unwired: 1 in]
        n290 = To Variant(anything=w507) -> (Variant=w498:variant)
        n291 = case shown="True" w441 {
          tunnel: ["Plot" ("Message") "Plot and Save" ("Message")] -> w499
          frame False {
          }
          frame True {
          }
        }
        n292 = Unbundle By Name(w438) -> ("Program status"=w415:string)
        n293 = case shown="\"INTERRUPTED\"" w415 {
          tunnel: [u32 16723242 u32 6618880 u32 16449369 u32 16449369 u32 16449369] -> w464
          frame "Stopped", Default {
          }
          frame "ACTIVE" {
          }
          frame "INTERRUPTED" {
          }
          frame "FEED_HOLD" {
          }
          frame "READY" {
          }
        }
        n294 = Bundle(cluster=w467, w464) -> (w468:cluster{u32, u32})  [unwired: 1 in]
        n295 = Insert Into Array(array=w465, index=0, new element #1=w468, new element #2=w468, new element #3=w468, new element #4=w468) -> (w466:cluster{u32, u32}[])
        n296 = property on="Property Node" class="Bool (strict)"(reference=w471, "Colors [4]"=w466) -> ()  [unwired: 1 in, 2 out]
        n297 = Equal?(x=w415, y="ACTIVE") -> (x = y?=w414:bool)
        n298 = Index Array(array=w478, index (row)=0, index (col)=0 ("disabled index (col)")) -> (element=w475:dbl)
        n299 = call "Enqueue Message.vi"("error in (no error)"=w500, "Message Data"=w498, "Message"=w499, "Message Queue"=w492) -> ("error out"=w472:errorcluster)  [unwired: 6 in, 1 out]
        n300 = call "UI Error Handler - Monitoring.vi"("error in (no error)"=w472, "Message Queue"=w523) -> ()  [unwired: 9 in, 1 out]
        n301 = Greater?(x=w475, y="In-cut Power Threshold") -> (0:w460:bool)
        n302 = And(x=w460, y=w441) -> (x .and. y?=w459:bool)
        n303 = case shown="False" w459 {
          tunnel: w434 -> [_ w557]
          tunnel: [w556 w557] -> w463
          tunnel: i16[] [0, 0, 0] ("0, 1") -> [w556 _]
          frame False {
          }
          frame True {
          }
        }
        n304 = Not Equal To 0?(x=w463) -> (x != 0?=w462:bool[])
        n305 = Or Array Elements(Boolean array=w462) -> (logical OR=→"Chatter?":bool)
        n306 = case shown="True" w414 {
          tunnel: [sgl 0.0 ("Tolerance") sgl 1.0 ("Tolerance")] -> w413
          tunnel: [FALSE TRUE] -> w411
          frame False {
          }
          frame True {
          }
        }
        n307 = Or(x=w412, y=w411) -> (x .or. y?=w410:bool)
        n308 = Bundle By Name(cluster=cluster{"Number of teeth":sgl} {"Number of teeth"=0.0} ("Tool data"), "Number of teeth"=w413) -> (w488:cluster{"Number of teeth":sgl})
        n309 = Bundle By Name(cluster=cluster{"G1 ":bool} {"G1 "=FALSE} ("G1 status"), "G1"=w410) -> (w452:cluster{"G1 ":bool})
        "output cluster" <- w452
        n310 = Bundle By Name(cluster=T9 {"Tool data"={"Number of teeth"=2.0}, "Cutting data"={"rpm"=9898.0}, "Limits"={"Magnitude threshold"=0.0, "Tolerance"=1.0}, "G1 status"={"G1 "=FALSE}} ("Chatter Data"), "Tool data"=w488, "Cutting data"=w486, "Limits"=w484, "G1 status"=w452) -> (w480:T9)
        n311 = call "Enqueue Message.vi"("Message Data"=w480, "Message"="Update Control Configuration", "Message Queue"=w492) -> ()  [unwired: 7 in, 2 out]
      }
    }
    n312 = global read "Global - All UI Loop Stop.vi" "All UI Loop Stop"() -> (w407:bool)
  }
  n313 = Unregister For Events(event registration refnum=w31, error in=w39) -> (error out=w32:errorcluster)
  n314 = Merge Errors(w32, w40) -> (w38:errorcluster)
  n315 = call "Destroy User Event - Stop.vi"("error in (no error)"=w38, "User Event - Stop"=w36) -> ("error out"=w30:errorcluster)  [unwired: 9 in]
  n316 = call <vilib>:"Simple Error Handler.vi"("error in (no error)"=w30) -> ()  [unwired: 4 in, 5 out]
